vi "LimitTo1.vi"(1 "Input":dbl) -> (0 "Output":dbl)   [LabVIEW 2015]
panel:
  # "Limit to [0,1]"
  # "This VI simply coerces the input value to be within [0,1] and then outputs the coerced value."
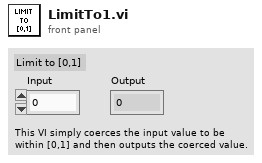
[diagram p1: front panel]
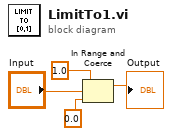
[diagram p0: block diagram]
diagram:
  n1 = In Range and Coerce(upper limit=1.0, x="Input", lower limit=0.0) -> (coerced(x)=→"Output":dbl)  [unwired: 1 out]
